vi "USRP Packet TX2.vi"() -> ()   [LabVIEW 2019]
uses:
  <instrlib>/niUSRP/niUSRP Write Tx Data (CDB Cluster).vi
  <vilib>/addons/Modulation/Digital/General/MT Generate PSK System Parameters(M).vi
  <vilib>/addons/Modulation/niDMT.lvlib
panel:
  out "Transmitted picture":picture
  in  "path to JPEG file":path
  in  "Modulation type":string(combo)="QPSK"
  in  "16-PSK System Parameters 2":T1={"Samples per Symbol"=8, "symbol map"=[], "Differential PSK"=enum."disable", "PSK type"=0} caption="16-PSK System Parameters" {"PSK type" items=["normal", "shifted", "offset"]; "symbol map" format="%.3f"}
  in  "8-PSK System Parameters 2":T1={"Samples per Symbol"=8, "symbol map"=[], "Differential PSK"=enum."disable", "PSK type"=0} caption="8-PSK System Parameters" {"PSK type" items=["normal", "shifted", "offset"]; "symbol map" format="%.3f"}
  in  "QPSK System Parameters 2":T1={"Samples per Symbol"=8, "symbol map"=[], "Differential PSK"=enum."disable", "PSK type"=0} caption="QPSK System Parameters" {"PSK type" items=["normal", "shifted", "offset"]; "symbol map" format="%.3f"}
  in  "BPSK System Parameters 2":T1={"Samples per Symbol"=8, "symbol map"=[], "Differential PSK"=enum."disable", "PSK type"=0} caption="BPSK System Parameters" {"PSK type" items=["normal", "shifted", "offset"]; "symbol map" format="%.3f"}
  in  "PN sequence order\nfor Sync Bits":i32=31 caption="PN sequence order (9)"
  in  "USRP IP address":refnum<k15>="192.168.10.2"
  in  "Packet Pad \n[samples]":i32=200
  out "Number of Packets in Message":i32=46
  in  "Message Type":bool=TRUE
  in  "Tx Parameters":T2={"Tx IQ Sampling\nRate [s/sec]"=400000.0, "Tx Frequency [Hz]"=915000000.0, "Tx Gain [dB]"=0.0, "Tx Antenna"="TX1"} {"Tx Gain [dB]" format="%#.6p"; "Tx Frequency [Hz]" format="%#.6p"; "Tx IQ Sampling\nRate [s/sec]" format="%#.6p"}
  out "Actual Tx Parameters":T2={"Tx IQ Sampling\nRate [s/sec]"=400000.0, "Tx Frequency [Hz]"=915000000.0, "Tx Gain [dB]"=0.0, "Tx Antenna"="TX1"} {"Tx Gain [dB]" format="%#.6p"; "Tx Frequency [Hz]" format="%#.6p"; "Tx IQ Sampling\nRate [s/sec]" format="%#.6p"}
  in  "Packet Parameters":T3={"Guard Bits "=30, "Sync Bits"=20, "Message Bits"=128}
  out "error out":errorcluster
  out "Constellation Graph":T4(graph)
  in  "autoscale":bool
  out "Transmitted Signal":cluster{"t0":dbl, "dt":dbl, "Y":dbl[]}(graph)
  in  "Queue Length":i32=10
  in  "Blank Frame \n[samples]":i32=500
  in  "Pulse Shaping Filter Parameters":T5={"Alpha"=0.5, "Filter Length"=6, "TX Filter"=enum."Root Raised Cos"} caption="Pulse Shaping Filter" {"Alpha" format="%.2f"}
  out "Symbol Rate [symbols/sec]":dbl=50000.0 format="%#.6p"
  in  "stop":bool
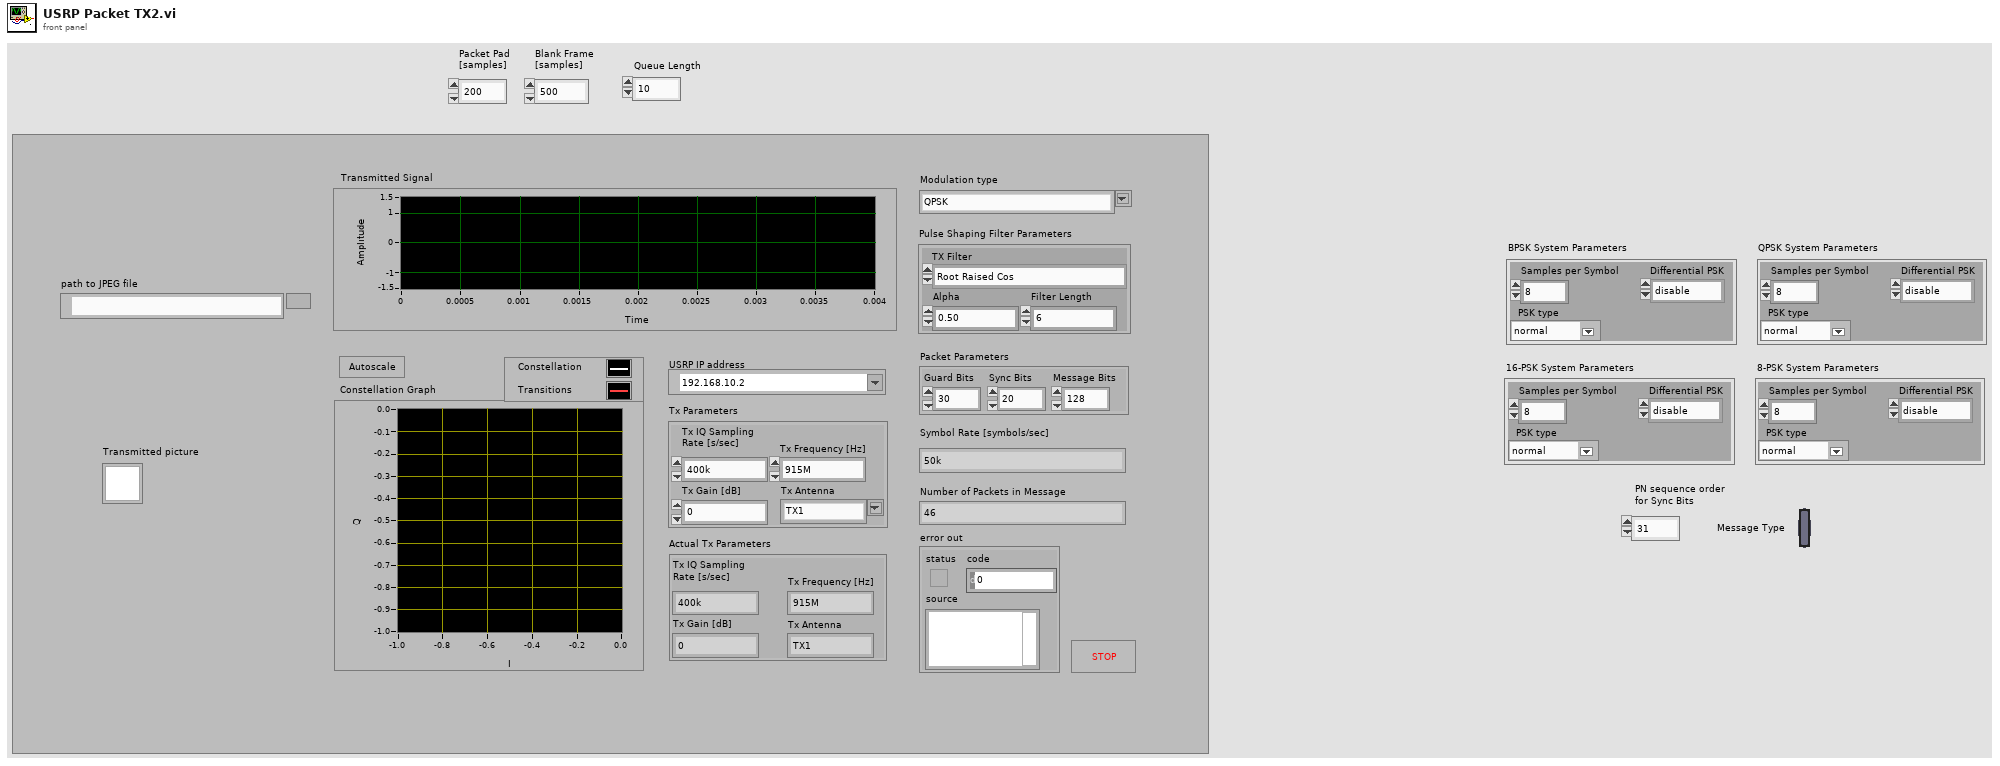
[diagram p1: front panel]
types:
  T1 = cluster{"Samples per Symbol":i32, "symbol map":cdb[], "Differential PSK":enum16{"disable", "enable"}, "PSK type":u16}
  T2 = cluster{"Tx IQ Sampling\nRate [s/sec]":dbl, "Tx Frequency [Hz]":dbl, "Tx Gain [dB]":dbl, "Tx Antenna":string}
  T3 = cluster{"Guard Bits ":i32, "Sync Bits":i32, "Message Bits":i32}
  T4 = cluster{"Decimated Array":dbl[], "Decimated Array":dbl[]}[]
  T5 = cluster{"Alpha":dbl, "Filter Length":i32, "TX Filter":enum16{"none", "Raised Cosine", "Root Raised Cos", "Gaussian"}}
  T6 = cluster{"samples per symbol (16)":i32, "symbol map":cdb[], "differential PSK":enum16{"disable", "enable"}, "PSK type":u16}
  T7 = cluster{"s? t:f":cluster{"t0":dbl, "dt":dbl, "Y":cdb[]}, i32}
  T8 = cluster{"output complex waveform":cluster{"t0":dbl, "dt":dbl, "Y":cdb[]}, i32}
  T9 = cluster{"constellation":dbl[], "oversampled data":dbl[]}[]
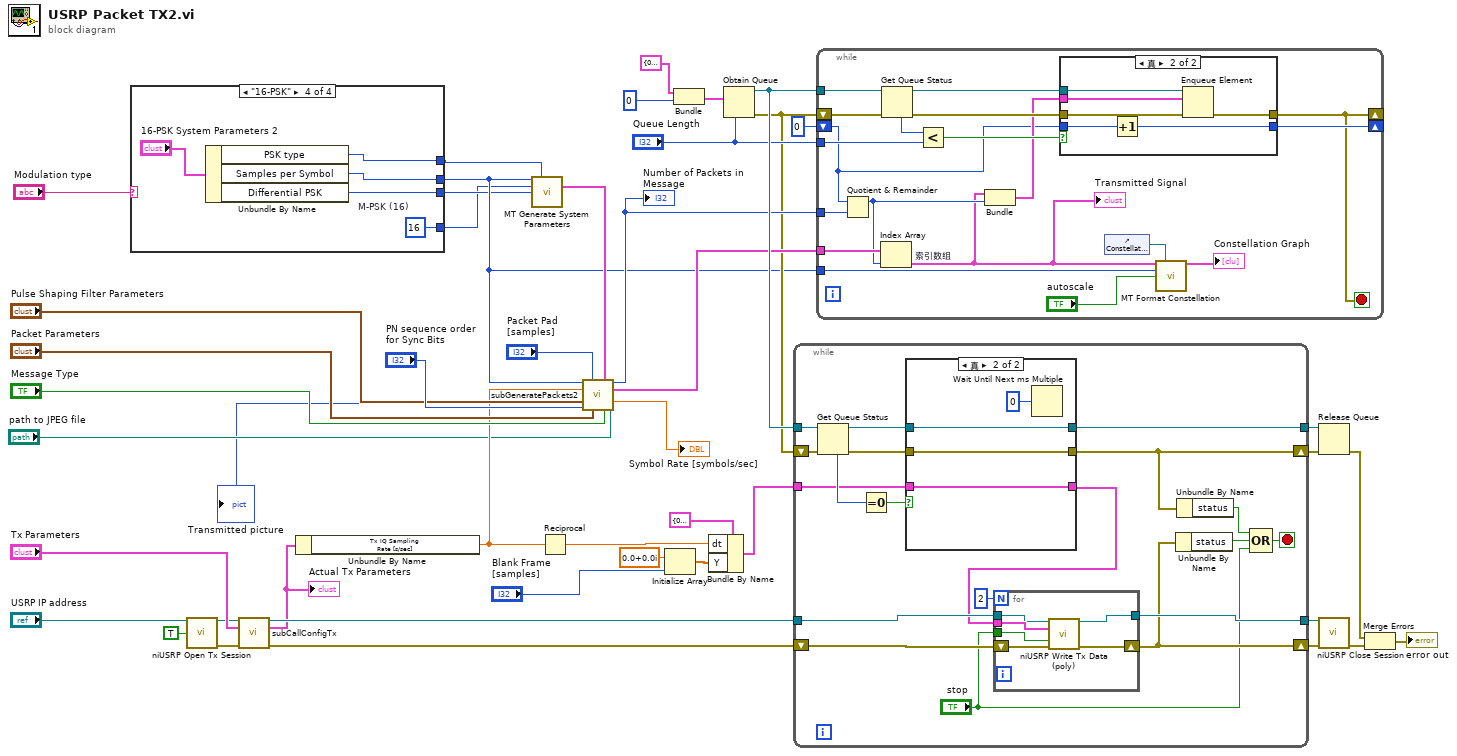
[diagram p0: block diagram]
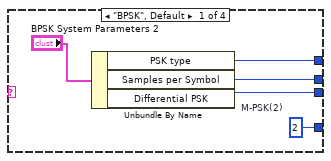
[diagram p2: hidden frame]
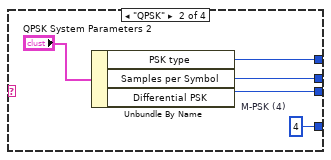
[diagram p3: hidden frame]
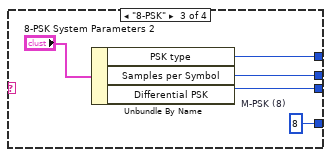
[diagram p4: hidden frame]
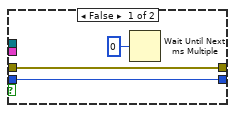
[diagram p5: hidden frame]
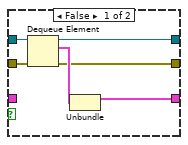
[diagram p6: hidden frame]
diagram:
  n1 = case shown="\"16-PSK\"" "Modulation type" {
    tunnel: [w47 w51 w59 w65] -> w5
    tunnel: [w48 w53 w58 w64] -> w4
    tunnel: [w50 w55 w57 w63] -> w3
    tunnel: [w49 w54 w60 w62] -> w6
    frame "BPSK", Default {
      w50 = 2  # M-PSK(2)
      n2 = Unbundle By Name("BPSK System Parameters 2") -> ("PSK type"=w49:u16, "Samples per Symbol"=w47:i32, "Differential PSK"=w48:enum16{"disable", "enable"})
    }
    frame "QPSK" {
      w55 = 4  # M-PSK (4)
      n3 = Unbundle By Name("QPSK System Parameters 2") -> ("PSK type"=w54:u16, "Samples per Symbol"=w51:i32, "Differential PSK"=w53:enum16{"disable", "enable"})
    }
    frame "8-PSK" {
      w57 = 8  # M-PSK (8)
      n4 = Unbundle By Name("8-PSK System Parameters 2") -> ("PSK type"=w60:u16, "Samples per Symbol"=w59:i32, "Differential PSK"=w58:enum16{"disable", "enable"})
    }
    frame "16-PSK" {
      w63 = 16  # M-PSK (16)
      n5 = Unbundle By Name("16-PSK System Parameters 2") -> ("PSK type"=w62:u16, "Samples per Symbol"=w65:i32, "Differential PSK"=w64:enum16{"disable", "enable"})
    }
  }
  n6 = call <instrlib>:"niUSRP Open Tx Session.vi"("device names"="USRP IP address", "reset"=TRUE) -> ("session handle out"=w20:refnum<k15>, "error out"=w19:errorcluster)  [unwired: 12 in]
  n7 = call "subCallConfigTx.vi"("session handle"=w20, "Tx Parameters"="Tx Parameters", "error in"=w19) -> ("session handle out"=w28:refnum<k15>, "Actual Tx Parameters"=w27:T2, "error out"=w32:errorcluster)  [unwired: 10 in]
  "Actual Tx Parameters" <- w27
  n8 = Unbundle By Name(w27) -> ("Tx IQ Sampling\nRate [s/sec]"=w10:dbl)
  n9 = call-poly <vilib>:"MT Generate System Parameters.vi"("samples per symbol (16)"=w5, "PSK type"=w6, "M-PSK (4)"=w3, "differential PSK"=w4) -> ("PSK system parameters"=w17:T6)  [unwired: 9 in, 2 out]
  n10 = Reciprocal(x=w10) -> (1/x=w29:dbl)
  n11 = call "subGeneratePackets2.vi"("Samples per Symbol"=w5, "Packet Pad \n[samples]"="Packet Pad \n[samples]", "PSK system parameters"=w17, "Tx IQ Sampling\nRate [s/sec]"=w10, "Pulse Shaping Filter Parameters"="Pulse Shaping Filter Parameters", "PN sequence order\nfor Sync Bits"="PN sequence order\nfor Sync Bits", "Packet Parameters"="Packet Parameters", "Message Type"="Message Type", "path to JPEG file"="path to JPEG file") -> ("Number of Packets"=w26:i32, "Packets"=w34:cluster{"t0":dbl, "dt":dbl, "Y":cdb[]}[], "Symbol Rate"=→"Symbol Rate [symbols/sec]":dbl, "Transmitted picture"=→"Transmitted picture":picture)  [unwired: 3 in]
  "Number of Packets in Message" <- w26
  n12 = Initialize Array(cdb 0.0+0.0i ("element"), "Blank Frame \n[samples]") -> (w42:cdb[])
  n13 = Bundle("s? t:f"=cluster{"t0":dbl, "dt":dbl, "Y":cdb[]} {"t0"=0.0, "dt"=0.0, "Y"=[]}, 0) -> (w37:T7)  [unwired: 1 in]
  n14 = Bundle By Name(cluster=cluster{"t0":dbl, "dt":dbl, "Y":cdb[]} {"t0"=0.0, "dt"=0.0, "Y"=[]} ("s? t:f"), "dt"=w29, "Y"=w42) -> (w41:cluster{"t0":dbl, "dt":dbl, "Y":cdb[]})
  n15 = Obtain Queue(max queue size (-1, unlimited)="Queue Length", element data type=w37) -> (queue out=w43:refnum<queue>, error out=w22:errorcluster)  [unwired: 3 in, 1 out]
  n16 = while {
    tunnel: w28 -> [w75]
    shift-right: [w72] -> w31
    shift-left: w32 -> [w76]
    tunnel: w43 -> [w84]
    tunnel: w41 -> [w81]
    tunnel: [w80] -> w40
    tunnel: [w74] -> w30
    shift-right: [w68] -> w39
    shift-left: w22 -> [w77]
    stop <- w71 stop-if-true
    n17 = Get Queue Status(queue=w84, error in (no error)=w77) -> (queue out=w79:refnum<queue>, error out=w78:errorcluster, # elements in queue=w83:i32)  [unwired: 1 in, 5 out]
    n18 = Equal To 0?(x=w83) -> (x = 0?=w82:bool)
    n19 = case shown="真" w82 {
      tunnel: w81 -> [_ w100]
      tunnel: [w92 w100] -> w66
      tunnel: [w96 w98] -> w80
      tunnel: [w91 w99] -> w68
      tunnel: w79 -> [w95 w98]
      tunnel: w78 -> [w94 w99]
      frame False {
        n20 = Dequeue Element(queue=w95, error in (no error)=w94) -> (queue out=w96:refnum<queue>, element=w93:T7, error out=w91:errorcluster)  [unwired: 1 in, 1 out]
        n21 = Unbundle(w93) -> ("s? t:f"=w92:cluster{"t0":dbl, "dt":dbl, "Y":cdb[]})  [unwired: 1 out]
      }
      frame True {
        n22 = Wait Until Next ms Multiple(millisecond multiple=u32 0) -> ()  [unwired: 1 out]
      }
    }
    n23 = for {
      N: 2 -> [_]
      tunnel: w66 -> [w89]
      tunnel: w75 -> [w88]
      tunnel: [w87] -> w74
      tunnel: "stop" -> [w86]
      shift-right: [w85] -> w72
      shift-left: w76 -> [w90]
      n24 = call-poly <instrlib>:"niUSRP Write Tx Data (poly).vi"("session handle"=w88, "data"=w89, "end of data?"=w86, "error in (no error)"=w90) -> ("session handle out"=w87:refnum<k15>, "error out"=w85:errorcluster)  [unwired: 10 in]
    }
    n25 = Unbundle By Name(w72) -> ("status"=w73:bool)
    n26 = Unbundle By Name(w68) -> ("status"=w67:bool)
    n27 = Compound Arithmetic op=OR(w67, w73, "stop") -> (w71:bool)
  }
  n28 = while {
    tunnel: w43 -> [w119]
    shift-right: [w112] -> _
    shift-left: 0 -> [w108]
    tunnel: w34 -> [w109]
    tunnel: "Queue Length" -> [w111]
    tunnel: w26 -> [w110]
    shift-right: [w106] -> _
    shift-left: w22 -> [w114]
    tunnel: w5 -> [w103]
    stop <- w106 stop-if-true
    n29 = Quotient & Remainder(x=w108, y=w110) -> (x-y*floor(x/y)=w107:i32)  [unwired: 1 out]
    n30 = Index Array "索引数组"(array=w109, index=w107) -> (element=w101:cluster{"t0":dbl, "dt":dbl, "Y":cdb[]})
    "Transmitted Signal" <- w101
    n31 = Get Queue Status(queue=w119, error in (no error)=w114) -> (queue out=w118:refnum<queue>, error out=w115:errorcluster, # elements in queue=w117:i32)  [unwired: 1 in, 5 out]
    n32 = Less?(x=w117, y=w111) -> (x < y?=w116:bool)
    n33 = Bundle("output complex waveform"=w101, w107) -> (w113:T8)  [unwired: 1 in]
    n34 = case shown="真" w116 {
      tunnel: w115 -> [w120 w128]
      tunnel: w118 -> [_ w127]
      tunnel: [w120 w126] -> w106
      tunnel: w113 -> [_ w125]
      tunnel: w108 -> [w122 w124]
      tunnel: [w122 w123] -> w112
      frame False {
        n35 = Wait Until Next ms Multiple(millisecond multiple=u32 0) -> ()  [unwired: 1 out]
      }
      frame True {
        n36 = Increment(x=w124) -> (x+1=w123:i32)
        n37 = Enqueue Element(queue=w127, element=w125, error in (no error)=w128) -> (error out=w126:errorcluster)  [unwired: 1 in, 2 out]
      }
    }
    n38 = control-ref of="Constellation Graph"() -> (w104:refnum<vi>)
    n39 = call <vilib>:"MT Format Constellation.vi"("waveform"=w101, "constellation reference"=w104, "samples per symbol"=w103, "autoscale"="autoscale") -> ("constellation graph"=→"Constellation Graph":T9)  [unwired: 1 in, 10 out]
  }
  n40 = Release Queue(queue=w40, error in (no error)=w39) -> (error out=w16:errorcluster)  [unwired: 3 out]
  n41 = call <instrlib>:"niUSRP Close Session.vi"("session handle"=w30, "error in (no error)"=w31) -> ("error out"=w15:errorcluster)  [unwired: 13 in]
  n42 = Merge Errors(w16, w15) -> (→"error out":errorcluster)
